vi "n_excess.vi"(4 "w":dbl, 5 "Vv":dbl, 6 "z":dbl, 7 "Vr":dbl, 8 "T":dbl, 9 "Pfp":dbl, 10 "Pf":dbl, 11 "Pi":dbl) -> (2 "nexcess":dbl)   [LabVIEW 2016]
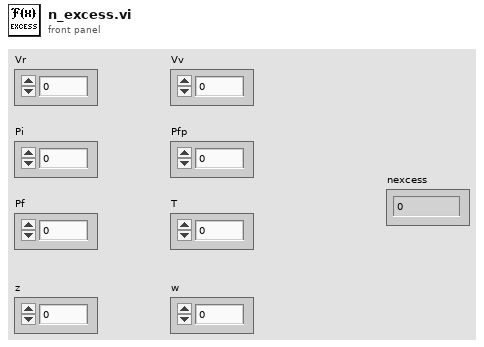
[diagram p1: front panel]
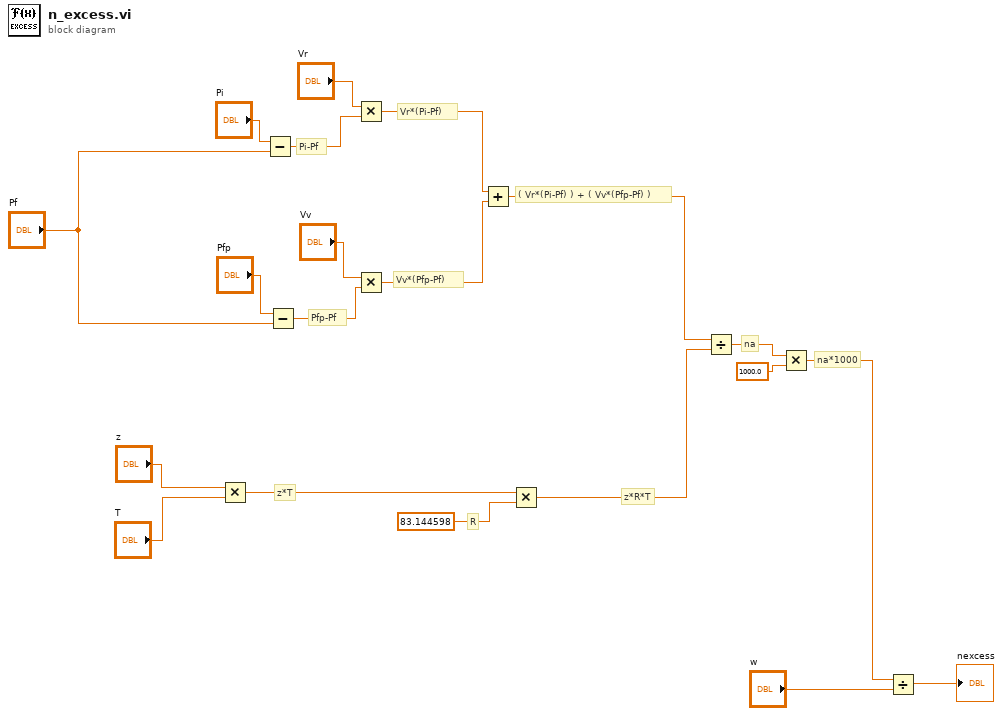
[diagram p0: block diagram]
diagram:
  # "Vv*(Pfp-Pf)"
  # "Vr*(Pi-Pf)"
  # "na*1000"
  # "na"
  # "z*T"
  # "z*R*T"
  # "( Vr*(Pi-Pf) ) + ( Vv*(Pfp-Pf) )"
  # "R"
  # "Pfp-Pf"
  # "Pi-Pf"
  n1 = Multiply(x="z", y="T") -> (x*y=w13:dbl)
  n2 = Subtract(x="Pi", y="Pf") -> (x-y=w20:dbl)
  n3 = Subtract(x="Pfp", y="Pf") -> (x-y=w19:dbl)
  n4 = Multiply(x="Vr", y=w20) -> (x*y=w18:dbl)
  n5 = Multiply(x="Vv", y=w19) -> (x*y=w17:dbl)
  n6 = Add(x=w18, y=w17) -> (x+y=w15:dbl)
  n7 = Multiply(x=w13, y=83.144598) -> (x*y=w14:dbl)
  n8 = Divide(x=w15, y=w14) -> (x/y=w12:dbl)
  n9 = Multiply(x=w12, y=1000.0) -> (x*y=w10:dbl)
  n10 = Divide(x=w10, y="w") -> (x/y=→"nexcess":dbl)
